vi "CtlsReplaced.vi"() -> ()   [LabVIEW 2016, in "SwitchDependenciesVariables.lvlib"]
uses:
  SwitchDependenciesVariables.lvlib
panel:
  in  "CtlsReplaced":string
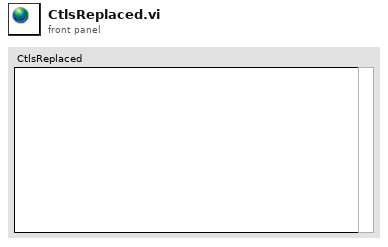
[diagram p1: front panel]
diagram:
